vi "Update Previous Button Visibility.vi"(8 "error in (no error)":errorcluster, 11 "Sensor Model in":refnum<class "Sensor Model.lvclass">) -> (0 "error out":errorcluster, 3 "Sensor Model out":refnum<class "Sensor Model.lvclass">)   [LabVIEW 2013, in "Sensor Model.lvlib" / "Sensor Model.lvclass"]
uses:
  Sensor Model.lvclass
  Sensor Model.lvclass/Sensor Model.ctl
  <vilib>/ActorFrameworkMVC/View Observer/View Registry/View Registry.lvclass/View Registry.ctl
  Sensor Model Messages/Abstract Sensor Previous Button Visibility Msg/Abstract Sensor Previous Button Visibility Msg.lvclass
  <vilib>/ActorFrameworkMVC/View Observer/Data Message/Data Message.lvclass
  <vilib>/ActorFrameworkMVC/View Observer/View Registry/View Registry.lvclass
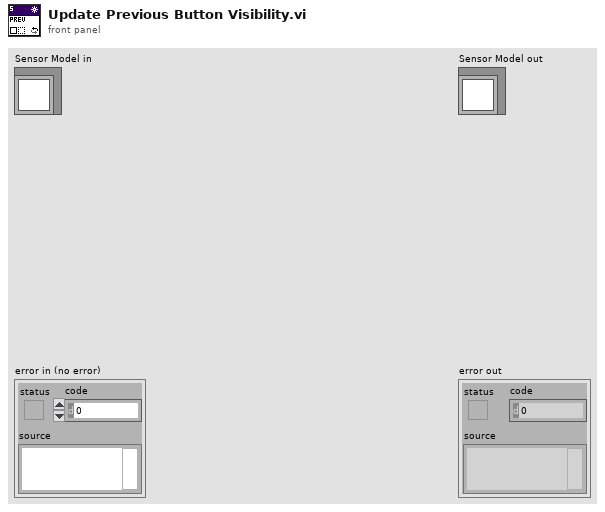
[diagram p1: front panel]
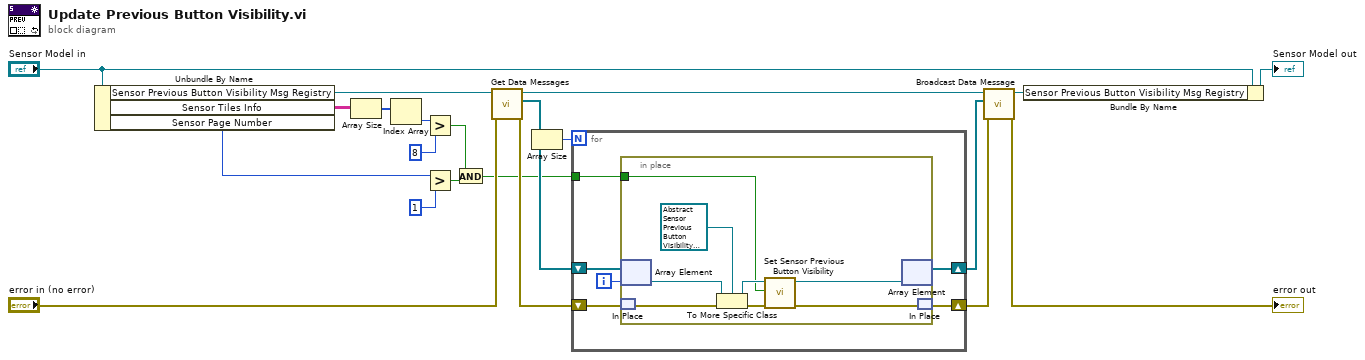
[diagram p0: block diagram]
diagram:
  n1 = Unbundle By Name("Sensor Model in") -> ("Sensor Previous Button Visibility Msg Registry"=w21:refnum<class "View Registry.lvclass">, "Sensor Tiles Info"=w3:string[][], "Sensor Page Number"=w2:i32)
  n2 = Array Size(array=w3) -> (size(s)=w8:i32[])
  n3 = Index Array(array=w8) -> (element=w5:i32)  [unwired: 1 in]
  n4 = Greater?(x=w5, y=8) -> (0:w7:bool)
  n5 = Greater?(x=w2, y=1) -> (0:w9:bool)
  n6 = And(x=w7, y=w9) -> (x .and. y?=w1:bool)
  n7 = call <vilib>:"Get Data Messages.vi"("error in (no error)"="error in (no error)", "View Registry in"=w21) -> ("error out"=w17:errorcluster, "Data Messages"=w18:refnum<class "Data Message.lvclass">[], "View Registry out"=w20:refnum<class "View Registry.lvclass">)  [unwired: 7 in]
  n8 = Array Size(array=w18) -> (size(s)=w19:i32)
  n9 = for {
    N: w19 -> [_]
    shift-right: [w26] -> w16
    shift-left: w18 -> [w27]
    shift-right: [w24] -> w15
    shift-left: w17 -> [w25]
    tunnel: w1 -> [w22]
    i -> [w23]
    n10 = in-place {
      in-place-border: w22 -> [w28]
      n11 = in-place-array #1(w27, w23) -> (w33:refnum<class "Data Message.lvclass">)
      n12 = in-place-match #2(w25) -> (w35:errorcluster)
      n13 = To More Specific Class(target class=refnum<class "Abstract Sensor Previous Button Visibility Msg.lvclass"> refnum ("Sensor Model.lvlib:Abstract Sensor Previous Button Visibility Msg.lvclass"), reference=w33, error in=w35) -> (specific class reference=w29:refnum<class "Abstract Sensor Previous Button Visibility Msg.lvclass">, error out=w32:errorcluster)
      n14 = call "Set Sensor Previous Button Visibility.vi"("error in (no error)"=w32, "Sensor Previous Button Visibility"=w28, "Abstract Sensor Previous Button Visibility Msg in"=w29) -> ("error out"=w31:errorcluster, "Abstract Sensor Previous Button Visibility Msg out"=w30:refnum<class "Abstract Sensor Previous Button Visibility Msg.lvclass">)  [unwired: 7 in]
      n15 = in-place-array #1(w30) -> (w26:refnum<class "Data Message.lvclass">[])  [unwired: 1 out]
      n16 = in-place-match #2(w31) -> (w24:errorcluster)
    }
  }
  n17 = call <vilib>:"Broadcast Data Message.vi"("error in (no error)"=w15, "Data Messages"=w16, "View Registry in"=w20) -> ("error out"=→"error out":errorcluster, "View Registry out"=w14:refnum<class "View Registry.lvclass">)  [unwired: 7 in]
  n18 = Bundle By Name(cluster="Sensor Model in", "Sensor Previous Button Visibility Msg Registry"=w14) -> (→"Sensor Model out":refnum<class "Sensor Model.lvclass">)
